vi "Read Child Window Data.vi"(8 "error in (no error)":errorcluster, 11 "LV Doc in":refnum<class "LV Doc.lvclass">) -> (0 "error out":errorcluster, 2 "Child Window Data":T1, 3 "LV Doc out":refnum<class "LV Doc.lvclass">)   [LabVIEW 2016, in "LV Doc.lvclass"]
uses:
  LV Doc.lvclass
  MDI Library/TypeDefs/Child Window Data.ctl
  LV Doc.lvclass/LV Doc.ctl
  MDI Library/LV MDI.lvclass
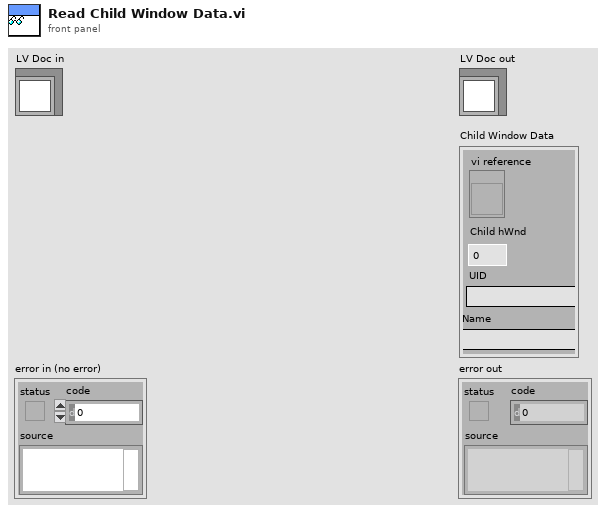
[diagram p1: front panel]
types:
  T1 = typedef "LV MDI.lvclass/Child Window Data.ctl" = cluster{"Child hWnd":u32, "UID":string, "vi reference":refnum<vi>, "Name":string}
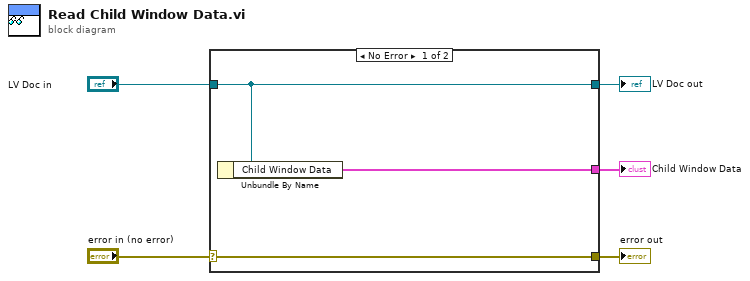
[diagram p0: block diagram]
diagram:
  n1 = case shown="No Error" "error in (no error)" {
    selector: "error in (no error)" -> [w8 w9]
    tunnel: [w8 w9] -> w4
    tunnel: [w7 w10] -> w2
    tunnel: "LV Doc in" -> [w7 w10]
    tunnel: [w6 _] -> w1
    frame No Error {
      n2 = Unbundle By Name(w7) -> ("Child Window Data"=w6:T1)
    }
    frame Error {
    }
  }
  "error out" <- w4
  "LV Doc out" <- w2
  "Child Window Data" <- w1
